vi "Read System Information.vi"(8 "error in (no error)":errorcluster, 11 "VISA resource name":refnum<visa-resource-name>) -> (0 "error out":errorcluster, 1 "Number of Ports":i32, 2 "Number of Traces":i32, 3 "VISA resource name out":refnum<visa-resource-name>, 4 "System Version":i32, 5 "Number of Channels":i32)   [LabVIEW 2011, in "Agilent ENA Series.lvlib"]
doc: "This VI reads system information."
uses:
  Agilent ENA Series.lvlib
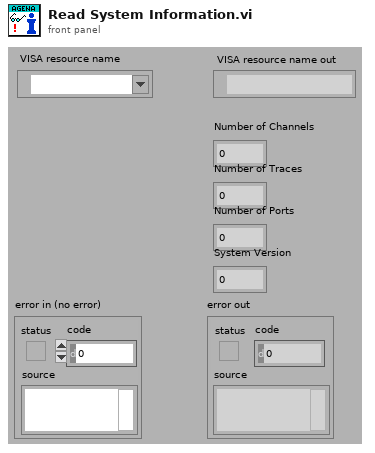
[diagram p1: front panel]
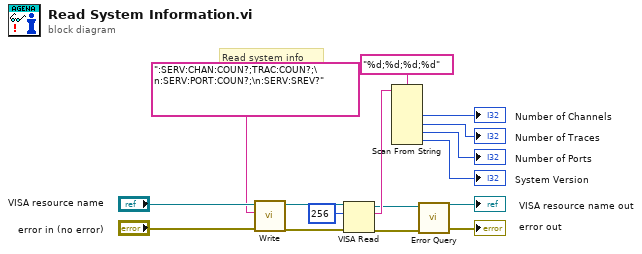
[diagram p0: block diagram]
diagram:
  # "Read system info"
  n1 = call "Write.vi"("error in (no error)"="error in (no error)", "String ()"=":SERV:CHAN:COUN?;TRAC:COUN?;\n:SERV:PORT:COUN?;\n:SERV:SREV?" ("format string"), "VISA resource name"="VISA resource name") -> ("error out"=w13:errorcluster, "VISA resource name out"=w12:refnum<visa-resource-name>)  [unwired: 6 in, 1 out]
  n2 = VISA Read(VISA resource name=w12, byte count=u32 256, error in (no error)=w13) -> (VISA resource name out=w1:refnum<visa-resource-name>, read buffer=w10:string, error out=w2:errorcluster)  [unwired: 1 out]
  n3 = Scan From String(format string="%d;%d;%d;%d", input string=w10) -> (output 1=→"Number of Channels":i32, output 2=→"Number of Traces":i32, output 3=→"Number of Ports":i32, output 4=→"System Version":i32)  [unwired: 6 in, 3 out]
  n4 = call "Error Query.vi"("error in (no error)"=w2, "VISA resource name"=w1) -> ("error out"=→"error out":errorcluster, "VISA resource name out"=→"VISA resource name out":refnum<visa-resource-name>)  [unwired: 6 in, 2 out]
